vi "Start Live Mode.vi"(8 "error in (no error)":errorcluster, 10 "Camera Settings":T1={"Exposure Time (ms)"=100.0, "Binning"=enum."2x2", "Scan Mode"=0, "Frames to Acquire"=1000.0, "Pixel Correction"=FALSE, "Frames to Skip"=0, "File Path"=path "", "Duty cycle"=0.0, "ALEX"=FALSE, "Shutter Enable"=[], "fluidics trigger frame"=0, "Bit Depth"=16, "Image Width (px)"=0, "Image Height (px)"=0, "Horizontal Offset (px)"=0, "Vertical Offset (px)"=0} {"fluidics trigger frame" max=60000 step=1; "Exposure Time (ms)" min=1.0 max=10000.0 step=1.0}, 11 "Camera in":refnum<class "Camera.lvclass">) -> (0 "error out":errorcluster, 3 "Camera out":refnum<class "Camera.lvclass">)   [LabVIEW 2023, in "Camera.lvlib" / "Camera.lvclass"]
uses:
  Camera.lvclass
  Camera.lvclass/Camera.ctl
  Resources/GLOBAL/GLOBAL Time-critical.vi
  <vilib>/ActorFramework/Actor/Actor.lvclass
  <vilib>/Utility/error.llb/DialogType.ctl
  Application Messages/Record Button Off Msg/Cancel Operation Msg.lvclass
  C:/Program Files/National Instruments/LabVIEW 2023/vi.lib/ActorFramework/Actor/Actor.lvclass
  Resources/Type Defs/Camera Settings.ctl
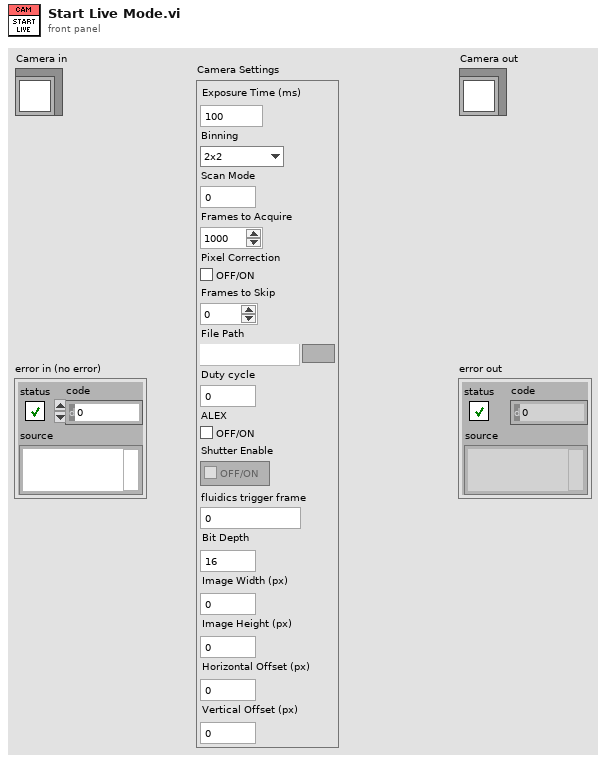
[diagram p1: front panel]
types:
  T1 = typedef "Camera Settings.ctl" = cluster{"Exposure Time (ms)":dbl, "Binning":enum16{"1x1", "2x2", "4x4"}, "Scan Mode":i32, "Frames to Acquire":dbl, "Pixel Correction":bool, "Frames to Skip":u32, "File Path":path, "Duty cycle":dbl, "ALEX":bool, "Shutter Enable":bool[], "fluidics trigger frame":u16, "Bit Depth":u16, "Image Width (px)":u16, "Image Height (px)":u16, "Horizontal Offset (px)":u16, "Vertical Offset (px)":u16}
  T2 = typedef "DialogType.ctl" = u16
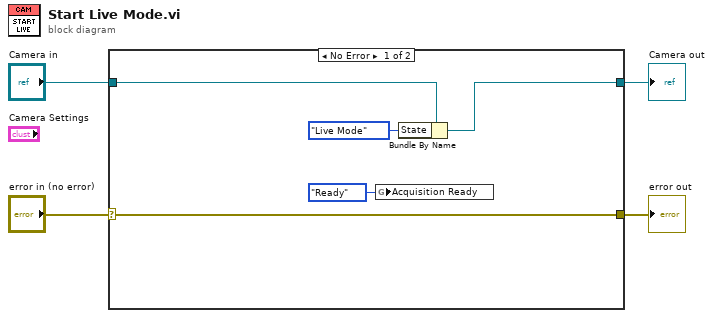
[diagram p0: block diagram]
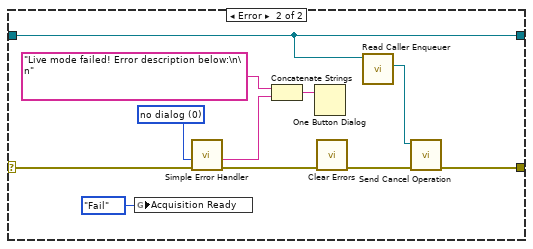
[diagram p2: hidden frame]
diagram:
  n1 = case shown="No Error" "error in (no error)" {
    selector: "error in (no error)" -> [w7 w20]
    tunnel: [w7 w12] -> w3
    tunnel: [w8 w19] -> w1
    tunnel: "Camera in" -> [w9 w19]
    frame No Error {
      n2 = global write "GLOBAL Time-critical.vi" "Acquisition Ready"(enum16{"Waiting", "Ready", "Fail", "Timeout"}."Ready" ("Acquisition Ready")) -> ()
      n3 = Bundle By Name(cluster=w9, "State"=enum16{"Idle", "Live Mode", "Streaming"}."Live Mode") -> (w8:refnum<class "Camera.lvclass">)
    }
    frame Error {
      w17 = T2 0 items=["no dialog", "OK message", "continue or stop message", "OK message + warnings", "continue/stop + warnings"] ("type of dialog (OK msg:1)")
      n4 = global write "GLOBAL Time-critical.vi" "Acquisition Ready"(enum16{"Waiting", "Ready", "Fail", "Timeout"}."Fail" ("Acquisition Ready")) -> ()
      n5 = call <vilib>:"Simple Error Handler.vi"("type of dialog (OK msg:1)"=w17, "error in (no error)"=w20) -> ("source out"=w15:string, "error out"=w18:errorcluster)  [unwired: 3 in, 3 out]
      n6 = Concatenate Strings("Live mode failed! Error description below:\n\n" ("string"), w15) -> (w16:string)
      n7 = One Button Dialog(message=w16) -> ()  [unwired: 1 in, 1 out]
      n8 = call <vilib>:"Clear Errors.vi"("error in (no error)"=w18) -> ("error out"=w13:errorcluster)  [unwired: 5 in, 1 out]
      n9 = call <vilib>:"Read Caller Enqueuer.vi"("Actor"=w19) -> ("Caller Enqueuer"=w11:refnum<class "Message Enqueuer.lvclass">)  [unwired: 10 in]
      n10 = call "Send Cancel Operation.vi"("error in (no error)"=w13, "Message Enqueuer"=w11) -> ("error out"=w12:errorcluster)  [unwired: 8 in, 1 out]
    }
  }
  "error out" <- w3
  "Camera out" <- w1
